vi "AltitudeIndicator.vi"(7 "GPS/Baro_Alt":bool, 8 "error in (no error)":errorcluster caption="Fehler (Eingang, kein Fehler)", 10 "MultiWii Data Cluster":T1 {"Altitude abs [m]" format="%.2f"; "Baro T [°C]" format="%.1f"; "Baro P [mbara]" format="%.1f"; "GPS_coord[LON]" format="%#_9f"; "GPS_coord[LAT]" format="%#_9f"; "Altitude [m]" format="%.2f"}, 11 "ScaleUnit(F=m; T=feet)":bool) -> (0 "error out":errorcluster caption="Fehler (Ausgang)", 2 "Altitude  (/10000)":dbl, 3 "AltitudeIndicator":picture, 4 "Altitude (ft)":string, 6 "Altitude (m)":string)   [LabVIEW 2017]
uses:
  IMU_Functions/IMU_Data_Cluster.ctl
  <vilib>/Utility/miscctls.llb/LVBoundsTypeDef.ctl
  <vilib>/picture/picture.llb/imagedata.ctl
panel:
  out "new picture":picture caption="Neue Grafik"
  # "switch control for altitude unit\nF = meter, T = feet"
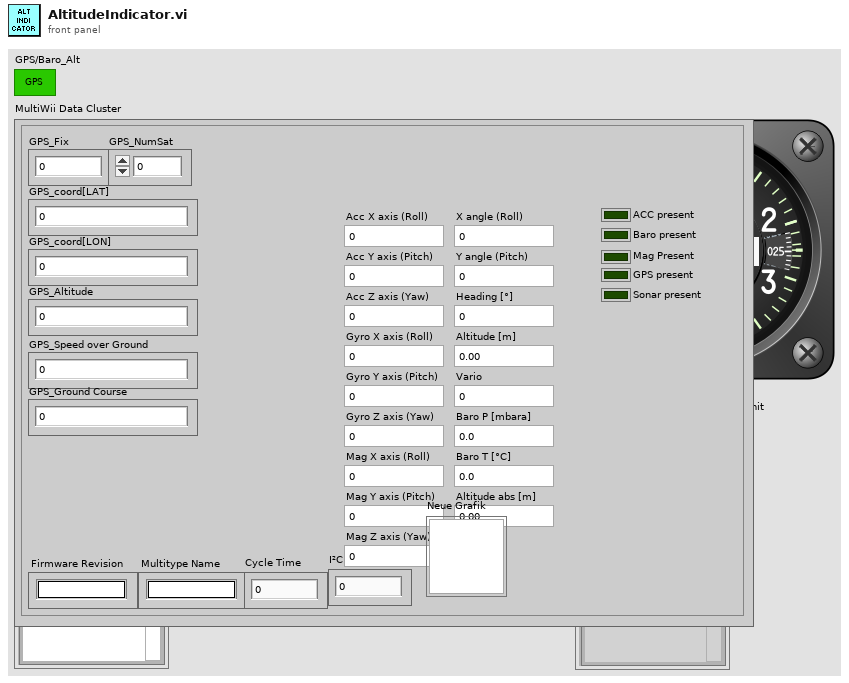
[diagram p1: front panel]
types:
  T1 = typedef "IMU_Data_Cluster.ctl" = cluster{"Firmware Revision":string, "Multitype Name":string, "Cycle Time":u16, "I²C Error Count":u16, "ACC present":bool, "Baro present":bool, "Mag Present":bool, "GPS present":bool, "Sonar present":bool, "Acc X axis (Roll)":dbl, "Acc Y axis (Pitch)":dbl, "Acc Z axis (Yaw)":dbl, "Gyro X axis (Roll)":dbl, "Gyro Y axis (Pitch)":dbl, "Gyro Z axis (Yaw)":dbl, "Mag X axis (Roll)":dbl, "Mag Y axis (Pitch)":dbl, "Mag Z axis (Yaw)":dbl, "X angle (Roll)":dbl, "Y angle (Pitch)":dbl, "Heading [°]":dbl, "Altitude [m]":dbl, "Vario":dbl, "GPS_Fix":u8, "GPS_NumSat":u8, "GPS_coord[LAT]":dbl, "GPS_coord[LON]":dbl, "GPS_Altitude":dbl, "GPS_Speed over Ground":dbl, "GPS_Ground Course":dbl, "Baro P [mbara]":dbl, "Baro T [°C]":dbl, "Altitude abs [m]":dbl}
  T2 = typedef "imagedata.ctl" = cluster{"image type":i32, "image depth":i32, "image":u8[], "mask":u8[], "colors":u32[], "Rectangle":cluster{"left":i16, "top":i16, "right":i16, "bottom":i16}}
  T3 = typedef "LVBoundsTypeDef.ctl" = cluster{"Width":u32, "Height":u32}
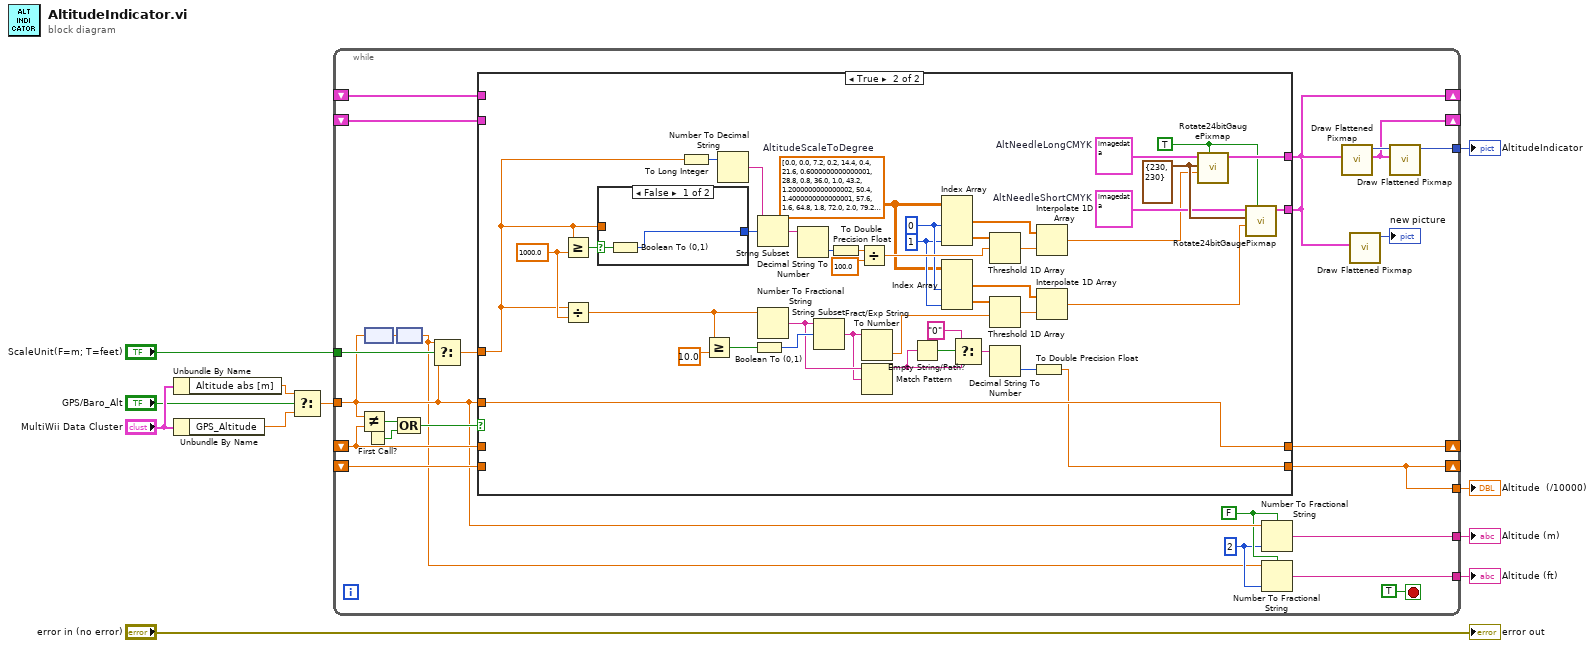
[diagram p0: block diagram]
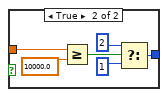
[diagram p3: hidden frame]
diagram:
  n1 = Unbundle By Name("MultiWii Data Cluster") -> ("Altitude abs [m]"=w2:dbl)
  n2 = Unbundle By Name("MultiWii Data Cluster") -> ("GPS_Altitude"=w3:dbl)
  n3 = Select(t=w2, s="GPS/Baro_Alt", f=w3) -> (s? t:f=w1:dbl)
  n4 = while {
    shift-right: [w33] -> _
    shift-left: _ -> [w30]
    shift-right: [w26] -> _
    shift-left: _ -> [w32]
    tunnel: [w25] -> w8
    tunnel: w1 -> [w19]
    shift-right: [w13] -> _
    shift-left: _ -> [w28]
    tunnel: "ScaleUnit(F=m; T=feet)" -> [w23]
    shift-right: [w20] -> _
    shift-left: _ -> [w21]
    tunnel: [w20] -> w7
    tunnel: [w15] -> w10
    tunnel: [w14] -> w9
    stop <- TRUE stop-if-true
    w18 = FALSE ("Systemdezimalzeichen verwenden (T)")
    w17 = i16 2 ("Genauigkeit (6)")
    n5 = Not Equal?(x=w19, y=w30) -> (x != y?=w34:bool)
    n6 = First Call?() -> (First Call?: T/F=w29:bool)
    n7 = node(w19) -> (w24:dbl[unit])
    n8 = node(w24) -> (w16:dbl)
    n9 = Compound Arithmetic op=OR(w34, w29) -> (w35:bool)
    n10 = Select(t=w16, s=w23, f=w19) -> (s? t:f=w22:dbl)
    n11 = case shown="True" w35 {
      tunnel: [w39 w81] -> w26
      tunnel: w32 -> [w39 _]
      tunnel: w30 -> [w38 _]
      tunnel: [w38 w44] -> w33
      tunnel: w19 -> [_ w44]
      tunnel: [w37 w80] -> w13
      tunnel: w28 -> [w37 _]
      tunnel: w22 -> [_ w41]
      tunnel: [w36 w40] -> w20
      tunnel: w21 -> [w36 _]
      frame False {
      }
      frame True {
        w48 = 1 ("Index (Spalte)")
        w49 = 0 ("Deaktivierter Index (Spalte)")
        w47 = dbl[][] [[0.0, 0.0], [7.2, 0.2], [14.4, 0.4], [21.6, 0.6000000000000001], [28.8, 0.8], [36.0, 1.0], [43.2, 1.2000000000000002], [50.4, 1.4000000000000001], [57.6, 1.6], [64.8, 1.8], [72.0, 2.0], [79.2, 2.2], [86.4, 2.4000000000000004], [93.60000000000001, 2.6], [100.8, 2.8000000000000003], [108.0, 3.0], [115.2, 3.2], [122.4, 3.4000000000000004], [129.6, 3.6], [136.8, 3.8000000000000003], [144.0, 4.0], [151.20000000000002, 4.2], [158.4, 4.4], [165.6, 4.6000000000000005], [172.8, 4.800000000000001], [180.0, 5.0], [187.20000000000002, 5.2], [194.4, 5.4], [201.6, 5.6000000000000005], [208.8, 5.800000000000001], [216.0, 6.0], [223.20000000000002, 6.2], [230.4, 6.4], [237.6, 6.6000000000000005], [244.8, 6.800000000000001], [252.0, 7.0], [259.2, 7.2], [266.40000000000003, 7.4], [273.6, 7.6000000000000005], [280.8, 7.800000000000001], [288.0, 8.0], [295.2, 8.200000000000001], [302.40000000000003, 8.4], [309.6, 8.6], [316.8, 8.8], [324.0, 9.0], [331.2, 9.200000000000001], [338.40000000000003, 9.4], [345.6, 9.600000000000001], [352.8, 9.8], [360.0, 10.0]]  # AltitudeScaleToDegree
        w45 = 1000.0 ("y")
        w76 = T2 {"image type"=0, "image depth"=24, "image"=array[158700 elements], "mask"=[], "colors"=[], "Rectangle"={"left"=0, "top"=0, "right"=230, "bottom"=230}}  # AltNeedleShortCMYK
        w77 = T2 {"image type"=0, "image depth"=24, "image"=array[158700 elements], "mask"=[], "colors"=[], "Rectangle"={"left"=0, "top"=0, "right"=230, "bottom"=230}}  # AltNeedleLongCMYK
        w78 = T3 {"Width"=230, "Height"=230} ("Größe des Darstellungsbereichs")
        w79 = TRUE ("Maske kombinieren? (F)")
        n12 = Greater Or Equal?(x=w41, y=w45) -> (x >= y?=w69:bool)
        n13 = Divide(x=w41, y=w45) -> (x/y=w62:dbl)
        n14 = case shown="False" w69 {
          selector: w69 -> [w83 _]
          tunnel: w41 -> [_ w88]
          tunnel: [w82 w84] -> w68
          frame False {
            n15 = Boolean To (0,1)(Boolean=w83) -> (0, 1=w82:i16)
          }
          frame True {
            n16 = Greater Or Equal?(x=w88, y=10000.0) -> (x >= y?=w87:bool)
            n17 = Select(t=i16 2 ("0, 1"), s=w87, f=i16 1 ("0, 1")) -> (s? t:f=w84:i16)
          }
        }
        n18 = To Long Integer(number=w41) -> (32bit integer=w72:i32)
        n19 = Greater Or Equal?(x=w62, y=10.0) -> (x >= y?=w66:bool)
        n20 = Number To Decimal String(number=w72) -> (decimal integer string=w75:string)  [unwired: 1 in]
        n21 = Boolean To (0,1)(Boolean=w66) -> (0, 1=w65:i16)
        n22 = String Subset(string=w75, offset (0)=w68) -> (substring=w74:string)  [unwired: 1 in]
        n23 = Number To Fractional String(number=w62) -> (F-format string=w64:string)  [unwired: 3 in]
        n24 = Decimal String To Number(string=w74) -> (number=w73:i32)  [unwired: 2 in, 1 out]
        n25 = String Subset(string=w64, offset (0)=w65) -> (substring=w63:string)  [unwired: 1 in]
        n26 = To Double Precision Float(number=w73) -> (double precision float=w70:dbl)
        n27 = Divide(x=w70, y=100.0) -> (x/y=w53:dbl)
        n28 = Fract/Exp String To Number(string=w63) -> (number=w46:dbl)  [unwired: 3 in, 1 out]
        n29 = Match Pattern(string=w64, regular expression=w63) -> (before substring=w60:string)  [unwired: 1 in, 3 out]
        n30 = Empty String/Path?(string/path=w60) -> (empty?=w61:bool)
        n31 = Index Array(array=w47, index (col) #1=w49, index (col) #2=w48) -> (element #1=w56:dbl[], element #2=w55:dbl[])  [unwired: 2 in]
        n32 = Index Array(array=w47, index (col) #1=w49, index (col) #2=w48) -> (element #1=w50:dbl[], element #2=w51:dbl[])  [unwired: 2 in]
        n33 = Select(t="0", s=w61, f=w60) -> (s? t:f=w57:string)
        n34 = Threshold 1D Array(2:w53, 3:w55) -> (0:w54:dbl)  [unwired: 1 in]
        n35 = Threshold 1D Array(2:w46, 3:w51) -> (0:w52:dbl)  [unwired: 1 in]
        n36 = Decimal String To Number(string=w57) -> (number=w58:i32)  [unwired: 2 in, 1 out]
        n37 = To Double Precision Float(number=w58) -> (double precision float=w40:dbl)
        n38 = Interpolate 1D Array(1:w54, 2:w56) -> (0:w43:dbl)
        n39 = Interpolate 1D Array(1:w52, 2:w50) -> (0:w42:dbl)
        n40 = call "Rotate24bitGaugePixmap.vi"("Maske kombinieren? (F)"=w79, "Rotation Angle (degrees)"=w43, "Größe des Darstellungsbereichs"=w78, "image data"=w77) -> ("image data out"=w81:T2)  [unwired: 7 in]
        n41 = call "Rotate24bitGaugePixmap.vi"("Maske kombinieren? (F)"=w79, "Rotation Angle (degrees)"=w42, "Größe des Darstellungsbereichs"=w78, "image data"=w76) -> ("image data out"=w80:T2)  [unwired: 7 in]
      }
    }
    n42 = Number To Fractional String(use system decimal point (T)=w18, number=w19, precision (6)=w17) -> (F-format string=w15:string)  [unwired: 1 in]
    n43 = Number To Fractional String(use system decimal point (T)=w18, number=w16, precision (6)=w17) -> (F-format string=w14:string)  [unwired: 1 in]
    n44 = call <vilib>:"Draw Flattened Pixmap.vi"("image data"=w13) -> ("new picture"=w27:picture)  [unwired: 1 in, 7 out]
    n45 = call <vilib>:"Draw Flattened Pixmap.vi"("image data"=w13) -> ("new picture"=→"new picture":picture)  [unwired: 8 in]
    n46 = call <vilib>:"Draw Flattened Pixmap.vi"("image data"=w26, "picture"=w27) -> ("new picture"=w25:picture)  [unwired: 7 out]
  }
  "Altitude (m)" <- w10
  "Altitude (ft)" <- w9
  "Altitude  (/10000)" <- w7
  "AltitudeIndicator" <- w8
  "error out" <- "error in (no error)"
